vi "Inficon - Read RealTime Thickness.vi"(8 "Error In":errorcluster, 11 "VISA in":refnum<visa-resource-name>) -> (0 "Error Out":errorcluster, 1 "RT Thickness":string, 2 "RT Thickness":dbl, 3 "VISA out":refnum<visa-resource-name>)   [LabVIEW 2014]
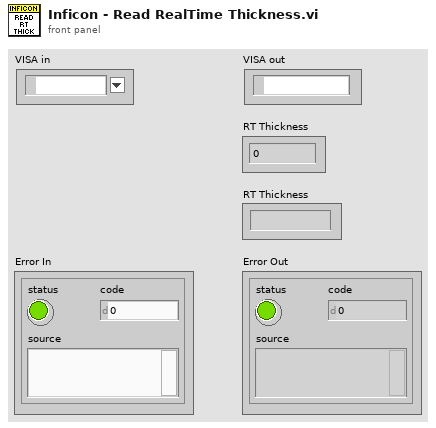
[diagram p1: front panel]
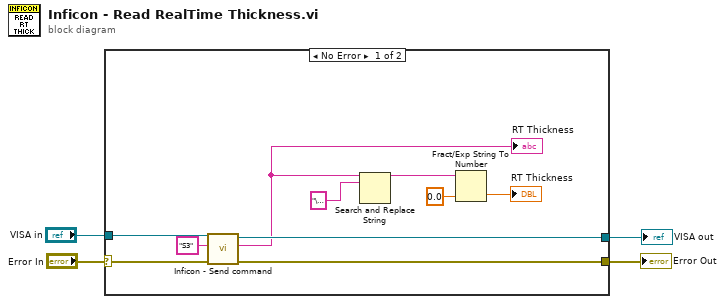
[diagram p0: block diagram]
diagram:
  n1 = case shown="No Error" "Error In" {
    selector: "Error In" -> [w14 w15]
    tunnel: [w13 w15] -> w3
    tunnel: "VISA in" -> [w12 w16]
    tunnel: [w10 w16] -> w1
    frame No Error {
      n2 = call "Inficon - Send command.vi"("Error In"=w14, "Command"="S3", "COM in"=w12) -> ("Error Out"=w13:errorcluster, "Output"=w5:string, "COM out"=w10:refnum<visa-resource-name>)  [unwired: 6 in]
      "RT Thickness" <- w5
      n3 = Search and Replace String(input string=w5, search string="\u0006") -> (result string=w7:string)  [unwired: 6 in, 3 out]
      n4 = Fract/Exp String To Number(string=w7, default (0 dbl)=0.0 ("default (0 I32)")) -> (number=→"RT Thickness":dbl)  [unwired: 2 in, 1 out]
    }
    frame Error {
    }
  }
  "Error Out" <- w3
  "VISA out" <- w1
